vi "Start.vi"(8 "error in (no error)":errorcluster, 11 "Mouse in":refnum<class "Mouse.lvclass">) -> (0 "error out":errorcluster, 3 "Mouse out":refnum<class "Mouse.lvclass">)   [LabVIEW 2020, in "Maze.lvlib" / "Mouse.lvclass"]
doc: "Start is called just before starting a new run. This allows reinitializing any class state as needed for the start of a run which is particularly useful if your mouse does any kind of internal mapping or route tracing."
uses:
  Mouse.lvclass
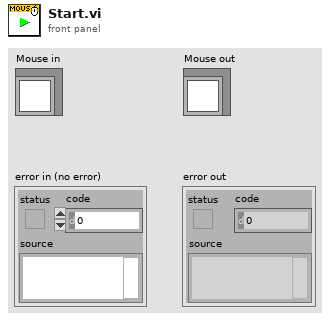
[diagram p1: front panel]
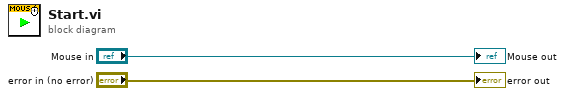
[diagram p0: block diagram]
diagram:
  "error out" <- "error in (no error)"
  "Mouse out" <- "Mouse in"
